vi "ACT_6_Task4_825005609.vi"() -> ()   [LabVIEW 2016]
panel:
  out "Waveform Chart 3":i32(graph)
  out "Waveform Chart 2":i32(graph)
  out "Waveform Chart":i32(graph)
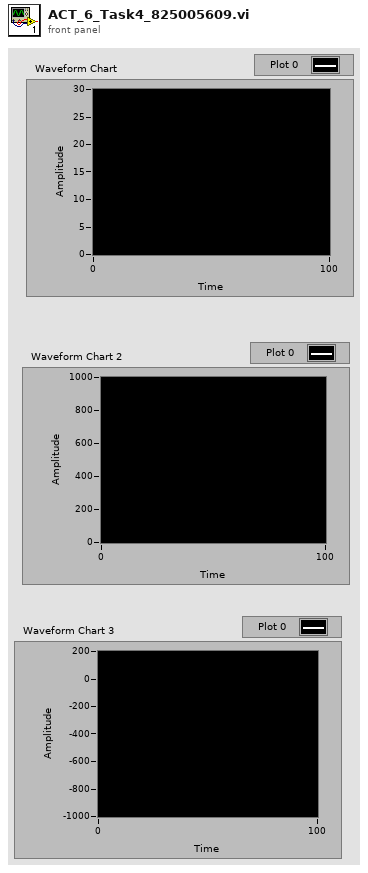
[diagram p1: front panel]
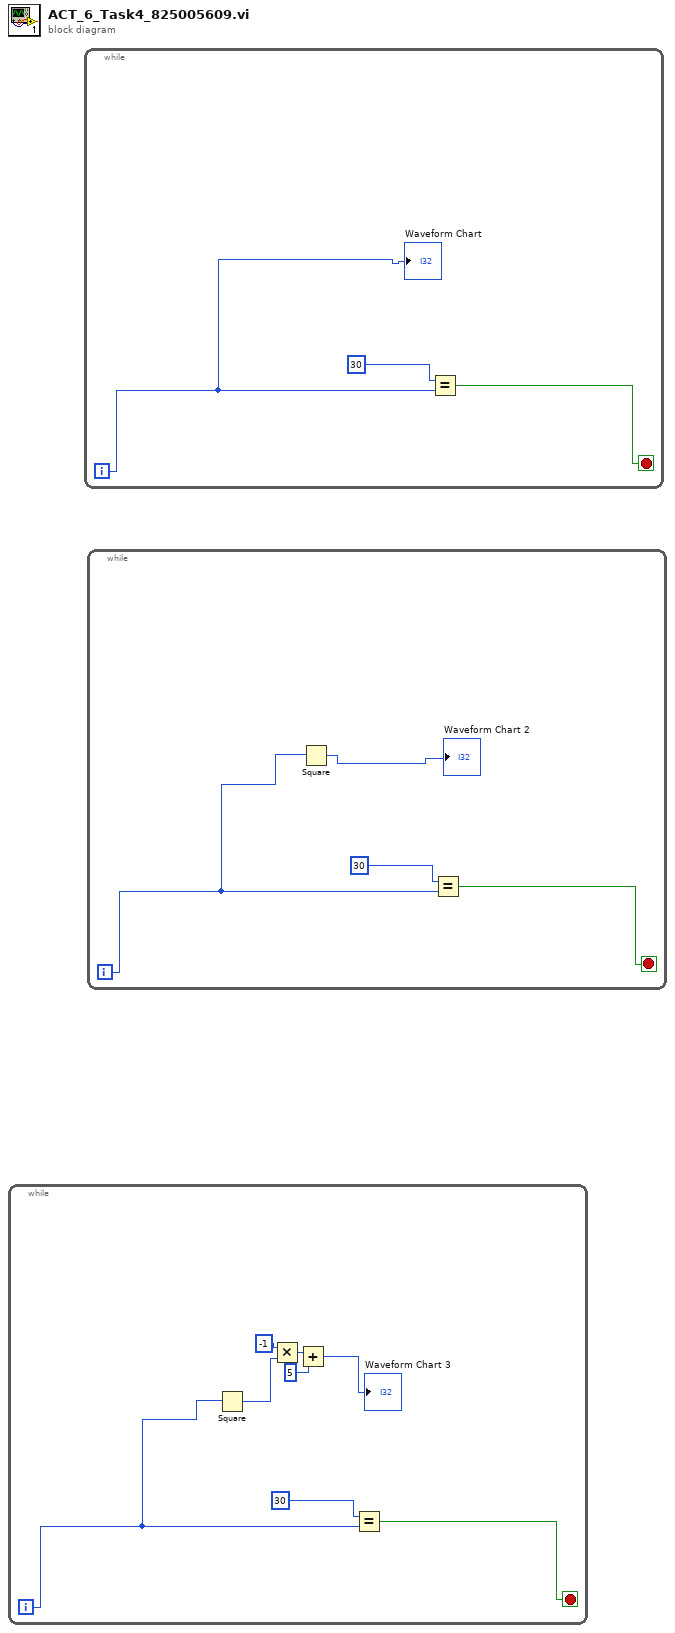
[diagram p0: block diagram]
diagram:
  n1 = while {
    i -> [w6]
    stop <- w8 stop-if-true
    n2 = Square(x=w6) -> (x^2=w4:i32)
    n3 = Multiply(x=-1, y=w4) -> (x*y=w5:i32)
    n4 = Add(x=w5, y=5) -> (x+y=→"Waveform Chart 3":i32)
    n5 = Equal?(x=30, y=w6) -> (x = y?=w8:bool)
  }
  n6 = while {
    i -> [w9]
    stop <- w11 stop-if-true
    n7 = Equal?(x=30, y=w9) -> (x = y?=w11:bool)
    "Waveform Chart" <- w9
  }
  n8 = while {
    i -> [w13]
    stop <- w15 stop-if-true
    n9 = Square(x=w13) -> (x^2=→"Waveform Chart 2":i32)
    n10 = Equal?(x=30, y=w13) -> (x = y?=w15:bool)
  }
